vi "TimeSyncAdjustTime.vi"(8 "error in":errorcluster, 10 "masterTime":timestamp, 11 "slaveTime":timestamp) -> (0 "error out":errorcluster)   [LabVIEW 2010]
uses:
  ts_custom.dll
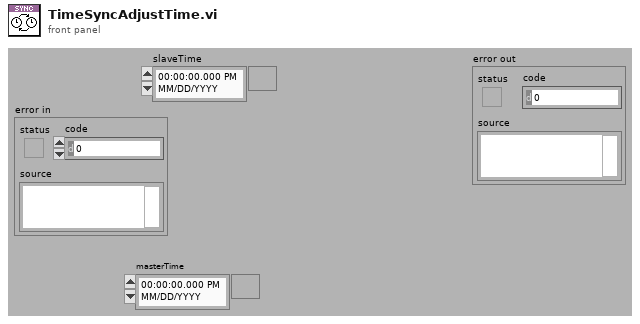
[diagram p1: front panel]
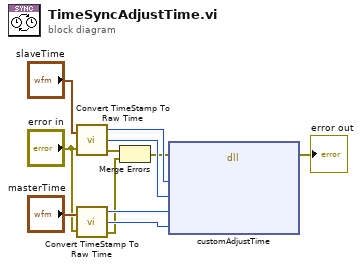
[diagram p0: block diagram]
diagram:
  n1 = call "Convert TimeStamp To Raw Time.vi"("error in (no error)"="error in", "time stamp"="slaveTime") -> ("error in (no error) 2"=w2:errorcluster, "Nanoseconds"=w8:u32, "Seconds"=w9:u32)
  n2 = call "Convert TimeStamp To Raw Time.vi"("error in (no error)"="error in", "time stamp"="masterTime") -> ("error in (no error) 2"=w3:errorcluster, "Nanoseconds"=w5:u32, "Seconds"=w6:u32)
  n3 = Merge Errors(w2, w3) -> (w1:errorcluster)
  n4 = dll-call lib="ts_custom.*" fn="customAdjustTime" ("ts_custom.*:integerAdjustTime")(error in=w1, "slaveTimeSeconds"=w9, "slaveTimeNanoseconds"=w8, "masterTimeSeconds"=w6, "masterTimeNanoseconds"=w5) -> (error out=→"error out":errorcluster)  [unwired: 7 in, 1 out]
